vi "Untitled 2.vi"() -> ()   [LabVIEW 2015, in "Untitled Library 1.lvlib"]
uses:
  Untitled Library 1.lvlib
panel:
  in  "stop":bool
  out "R1":u16
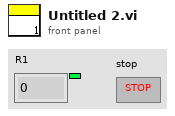
[diagram p1: front panel]
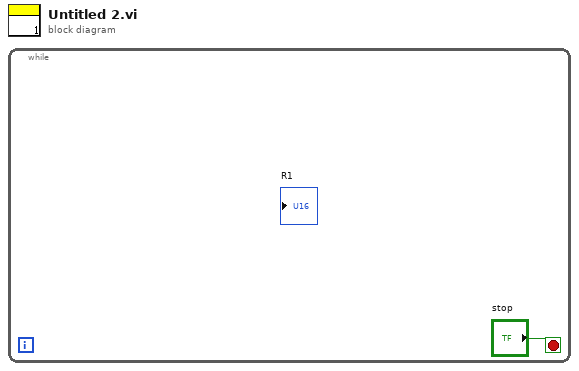
[diagram p0: block diagram]
diagram:
  n1 = while {
    stop <- "stop" stop-if-true
  }
